vi "Find Specification Match.vi"(7 "error in (no error)":errorcluster, 8 "Channel List":string[](array[string]), 10 "file path (dialog if empty)":path) -> (0 "error out":errorcluster, 1 "IVI Specifications":string[][](array[string]), 3 "Channel Specs":string[][](array[string]))   [LabVIEW 2019]
uses:
  <vilib>/Utility/file.llb/Read Delimited Spreadsheet (string).vi
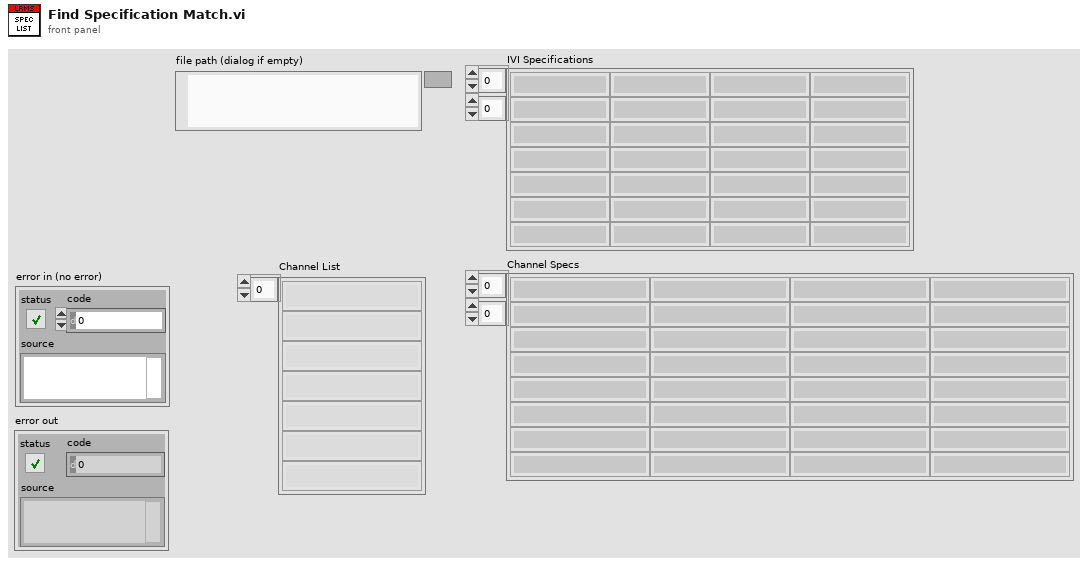
[diagram p1: front panel]
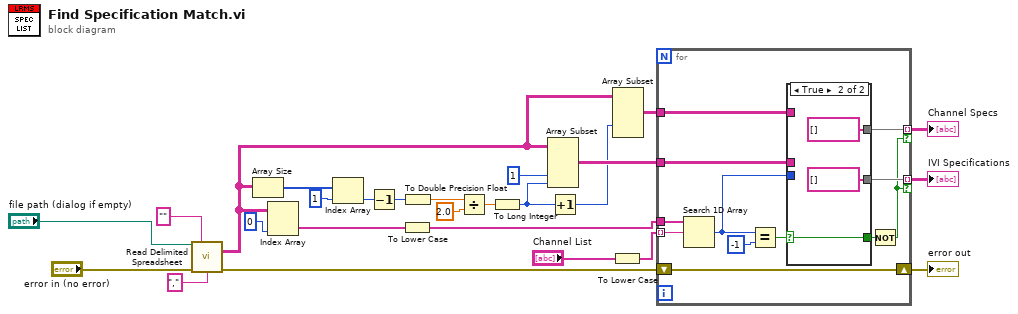
[diagram p0: block diagram]
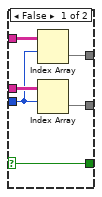
[diagram p2: hidden frame]
diagram:
  n1 = call-poly <vilib>:"Read Delimited Spreadsheet.vi"("file path (dialog if empty)"="file path (dialog if empty)", "format (%s)"="" ("format (%.3f)"), "error in (no error)"="error in (no error)", "delimiter (\\t)"="," ("delimiter (\\t)")) -> ("all rows"=w4:string[][], "error out"=w16:errorcluster)  [unwired: 6 in, 4 out]
  n2 = Array Size(array=w4) -> (size(s)=w15:i32[])
  n3 = Index Array(array=w4, index (col)=0 ("disabled index (col)")) -> (element=w2:string[])  [unwired: 1 in]
  n4 = Index Array(array=w15, index=1) -> (element=w13:i32)
  n5 = Decrement(x=w13) -> (x-1=w12:i32)
  n6 = To Lower Case(string=w2) -> (all lower case string=w5:string[])
  n7 = To Double Precision Float(number=w12) -> (double precision float=w8:dbl)
  n8 = Divide(x=w8, y=2.0) -> (x/y=w11:dbl)
  n9 = To Long Integer(number=w11) -> (32bit integer=w10:i32)
  n10 = Array Subset(array=w4, index (col)=1 ("index"), length (col)=w10) -> (w20:string[][])  [unwired: 2 in]
  n11 = Increment(x=w10) -> (x+1=w9:i32)
  n12 = To Lower Case(string="Channel List") -> (all lower case string=w6:string[])
  n13 = Array Subset(array=w4, index (col)=w9) -> (w21:string[][])  [unwired: 3 in]
  n14 = for {
    tunnel: w6 -> [w38] mode=indexing
    tunnel: w21 -> [w37]
    tunnel: [w36] -> w19 mode=indexing if=w27
    tunnel: w20 -> [w35]
    tunnel: [w30] -> w18 mode=indexing if=w27
    tunnel: w5 -> [w28]
    shift-right: [w34] -> w17
    shift-left: w16 -> [w34]
    n15 = Search 1D Array(1D array=w28, element=w38) -> (index of element=w33:i32)  [unwired: 1 in]
    n16 = Equal?(x=w33, y=-1) -> (x = y?=w31:bool)
    n17 = case shown="True" w31 {
      selector: w31 -> [w39 w45]
      tunnel: w37 -> [w44 _]
      tunnel: [w43 string[] []] -> w36
      tunnel: w35 -> [w42 _]
      tunnel: [w41 string[] []] -> w30
      tunnel: w33 -> [w40 _]
      tunnel: [w39 w45] -> w29
      frame False {
        n18 = Index Array(array=w44, index (row)=w40) -> (element=w43:string[])  [unwired: 1 in]
        n19 = Index Array(array=w42, index (row)=w40) -> (element=w41:string[])  [unwired: 1 in]
      }
      frame True {
      }
    }
    n20 = Not(x=w29) -> (.not. x?=w27:bool)
  }
  "Channel Specs" <- w19
  "IVI Specifications" <- w18
  "error out" <- w17
